vi "XY Graph Change Cursor Color.vi"(8 "Error In":errorcluster, 9 "Changed Color Index":i32, 10 "Changed Color":u32, 11 "XYGraph in":refnum<vi>) -> (0 "Error Out":errorcluster)   [LabVIEW 2021, in "XY Graph Add-Ons.lvlib"]
uses:
  XY Graph Add-Ons.lvlib
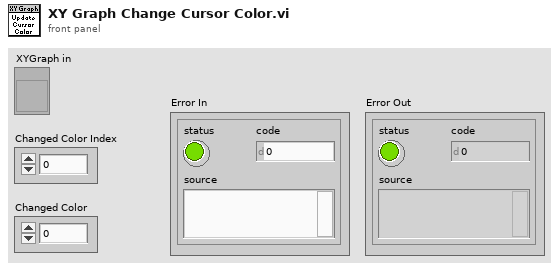
[diagram p1: front panel]
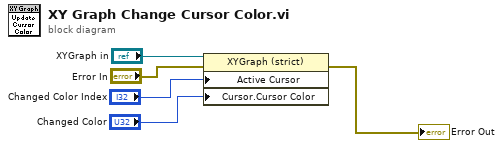
[diagram p0: block diagram]
diagram:
  n1 = property class="XYGraph (strict)"(reference="XYGraph in", error in="Error In", "Active Cursor"="Changed Color Index", "Cursor.Cursor Color"="Changed Color") -> (error out=→"Error Out":errorcluster)  [unwired: 1 out]
